vi "onAssertionSlippage.vi"(7 "AssertEqualValue in":refnum<class "AssertAlmostEqualValue.lvclass">, 10 "Properties":refnum<class "Properties.Assert.lvclass">) -> (0 "error out":errorcluster, 2 "Properties out":refnum<class "Properties.Assert.lvclass">)   [LabVIEW 2021, in "Bananas.lvlib" / "AssertAlmostEqualValue.lvclass"]
uses:
  AssertAlmostEqualValue.lvclass
  AssertAlmostEqualValue.lvclass/AssertAlmostEqualValue.ctl
  <vilib>/addons/_JKI Toolkits/Caraya/classes/Properties.Assert/Properties.Assert.lvclass
  <vilib>/addons/_JKI Toolkits/Caraya/classes/Properties/Properties.lvclass
  C:/Program Files (x86)/National Instruments/LabVIEW 2021/vi.lib/addons/_JKI Toolkits/Caraya/classes/Properties/Properties.lvclass
  C:/Program Files (x86)/National Instruments/LabVIEW 2021/vi.lib/addons/_JKI Toolkits/Caraya/classes/Properties.Assert/Properties.Assert.lvclass
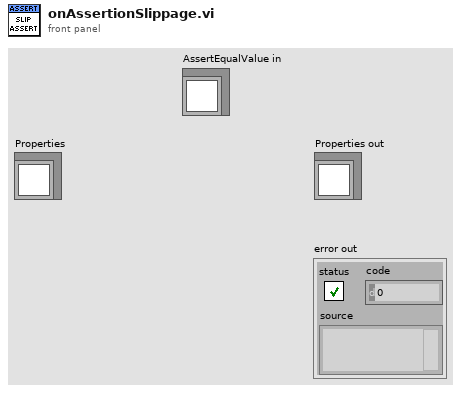
[diagram p1: front panel]
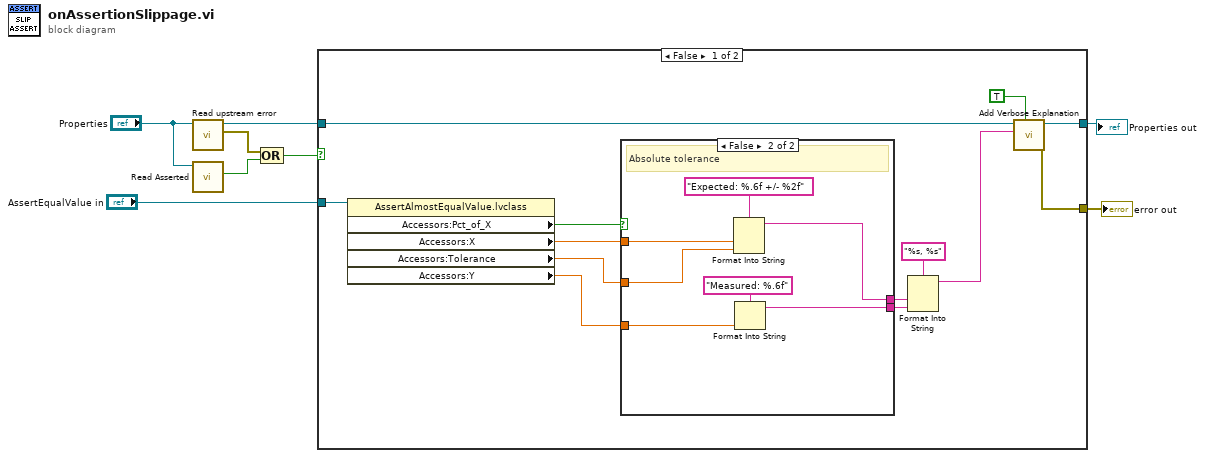
[diagram p0: block diagram]
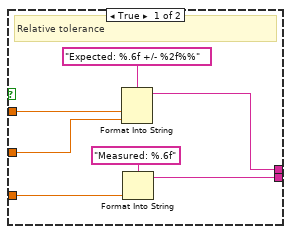
[diagram p2: hidden frame]
diagram:
  n1 = call <vilib>:"Read upstream error.vi"("Properties.Assert in"="Properties") -> ("upstream-error"=w7:errorcluster, "Properties.Assert out"=w8:refnum<class "Properties.Assert.lvclass">)  [unwired: 9 in]
  n2 = call <vilib>:"Read Asserted.vi"("Properties.Assert in"="Properties") -> ("Asserted"=w6:bool)  [unwired: 9 in, 1 out]
  n3 = Compound Arithmetic op=OR(w7, w6) -> (w5:bool)
  n4 = case shown="False" w5 {
    tunnel: [w20 w36] -> w3
    tunnel: [w19 _] -> w2
    tunnel: w8 -> [w21 w36]
    tunnel: "AssertEqualValue in" -> [w17 _]
    frame False {
      n5 = property class="AssertAlmostEqualValue.lvclass"(reference=w17) -> ("Accessors:Pct_of_X"=w12:bool, "Accessors:X"=w11:ext, "Accessors:Tolerance"=w9:ext, "Accessors:Y"=w10:ext)  [unwired: 1 in, 2 out]
      n6 = case shown="False" w12 {
        tunnel: [w27 w34] -> w15
        tunnel: [w25 w32] -> w14
        tunnel: w11 -> [w23 w30]
        tunnel: w10 -> [w24 w31]
        tunnel: w9 -> [w22 w29]
        frame True {
          # "Relative tolerance"
          n7 = Format Into String(format string="Expected: %.6f +/- %2f%%", w23, w22) -> (resulting string=w27:string)  [unwired: 2 in, 1 out]
          n8 = Format Into String(format string="Measured: %.6f", w24) -> (resulting string=w25:string)  [unwired: 2 in, 1 out]
        }
        frame False {
          # "Absolute tolerance"
          n9 = Format Into String(format string="Expected: %.6f +/- %2f", w30, w29) -> (resulting string=w34:string)  [unwired: 2 in, 1 out]
          n10 = Format Into String(format string="Measured: %.6f", w31) -> (resulting string=w32:string)  [unwired: 2 in, 1 out]
        }
      }
      n11 = Format Into String(format string="%s, %s", w15, w14) -> (resulting string=w13:string)  [unwired: 2 in, 1 out]
      n12 = call <vilib>:"Add Verbose Explanation.vi"("overwrite?"=TRUE, "Verbose Explanation"=w13, "Properties"=w21) -> ("error out"=w19:errorcluster, "Properties"=w20:refnum<class "Properties.Assert.lvclass">)  [unwired: 7 in]
    }
    frame True {
      # "There was an upstream error or the assertion = TRUE"
    }
  }
  "error out" <- w2
  "Properties out" <- w3
